vi "Check Variant Type.vi"(8 "error in (no error)":errorcluster, 10 "Variant":variant, 11 "String Value in":refnum<class "String Value.lvclass">) -> (0 "error out":errorcluster, 3 "String Value out":refnum<class "String Value.lvclass">)   [LabVIEW 2020]
uses:
  String Value.lvclass
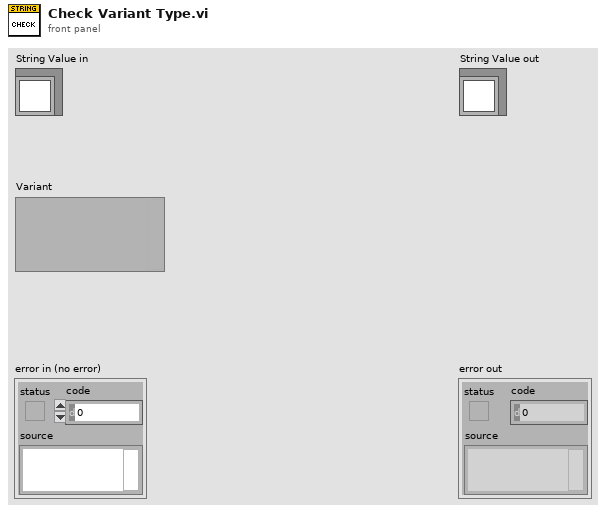
[diagram p1: front panel]
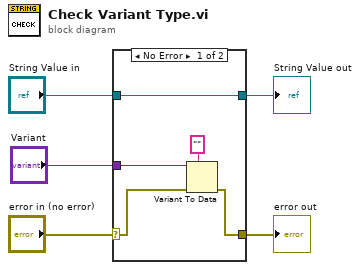
[diagram p0: block diagram]
diagram:
  n1 = case shown="No Error" "error in (no error)" {
    selector: "error in (no error)" -> [w6 w12]
    tunnel: [w8 w12] -> w4
    tunnel: "String Value in" -> [w9 w11]
    tunnel: [w9 w11] -> w2
    tunnel: "Variant" -> [w7 _]
    frame No Error {
      n2 = Variant To Data(error in=w6, type="", Variant=w7) -> (error out=w8:errorcluster)  [unwired: 1 out]
    }
    frame Error {
    }
  }
  "error out" <- w4
  "String Value out" <- w2
